vi "User Console View.vi"(8 "error in (no error)":errorcluster, 11 "View Model":T1) -> (0 "error out":errorcluster)   [LabVIEW 2017]
doc: "Provide processing user interaction with Elevator Controller by GUI controls."
uses:
  View Model/Controls/View Model.ctl
  Configuration/Controls/Config Model.ctl
  Configuration/Controls/Config Data.ctl
  Error Handler/Controls/Error Model.ctl
  Error Handler/Controls/Error Data.ctl
  Error Handler/Controls/Error Type.ctl
  View Model/Controls/Shared Model.ctl
  Elevator Controller/Controls/Elevator Model.ctl
  Elevator Controller/Controls/Elevator Location.ctl
  Elevator Controller/Controls/Elevator CMD Data.ctl
  Elevator Controller/Controls/Elevator Commands.ctl
  Elevator Controller/Controls/Elevator Overhead.ctl
  Elevator Controller/Controls/Elevator States.ctl
  Controls/User Console.ctl
panel:
  in  "Emergency":bool
  in  "1st Floor":bool
  in  "2nd Floor":bool
  in  "3rd Floor":bool
  in  "4th Floor":bool
  in  "Close Door":bool
  in  "Open Door":bool
  in  "Down 4":bool
  in  "Down 3":bool
  in  "Down 2":bool
  in  "Up 3":bool
  in  "Up 2":bool
  in  "Up 1":bool
  # "[Covers: UI1]"
  # "Floor Selection"
  # "Elevator Call"
  # "[Covers: UI2B]"
  # "[Covers: UI2A]"
  # "[Covers UI2A1]"
  # "[Covers UI2A2]"
  # "[Covers UI2B2]"
  # "by controls mechanical actions"
  # "[Covers: UI2C]"
  # "[Covers: UI2D]"
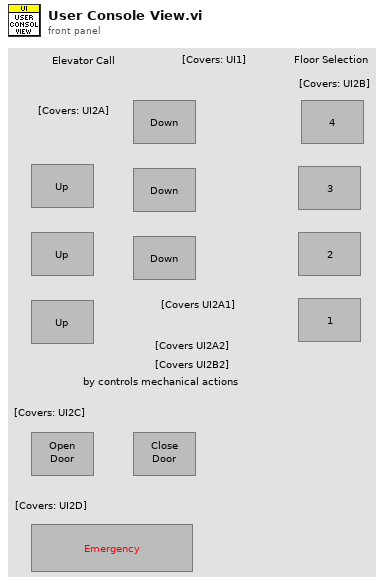
[diagram p1: front panel]
types:
  T1 = typedef "View Model.ctl" = cluster{"Config Model":T2, "Error Model":T3, "Shared Model":T4, "Elevator Model":T5}
  T2 = typedef "Config Model.ctl" = cluster{"Config Change":refnum<user-event>, "Config DVR":refnum<data-value>}
  T3 = typedef "Error Model.ctl" = cluster{"Error Event":refnum<user-event>}
  T4 = typedef "Shared Model.ctl" = cluster{"Stop Event":refnum<user-event>, "Stop DVR":refnum<data-value>}
  T5 = typedef "Elevator Model.ctl" = cluster{"Motion Change":refnum<user-event>, "Floor Change":refnum<user-event>, "Emergency Change":refnum<user-event>, "Direction Change":refnum<user-event>, "Door Position Change":refnum<user-event>, "Elevator CMD":refnum<user-event>, "Controller DVR":refnum<data-value>}
  T6 = typedef "User Console.ctl" = cluster{"Down 2":refnum<vi>, "Down 3":refnum<vi>, "Down 4":refnum<vi>, "Up 1":refnum<vi>, "Up 2":refnum<vi>, "Up 3":refnum<vi>, "1st Floor":refnum<vi>, "2nd Floor":refnum<vi>, "3rd Floor":refnum<vi>, "4th Floor":refnum<vi>, "Open Door":refnum<vi>, "Close Door":refnum<vi>, "Emergency":refnum<vi>}
  T7 = typedef "Elevator Commands.ctl" = enum16{"Go Up", "Go Down", "Go to Floor", "Open Doors", "Close Doors", "Emergency"}
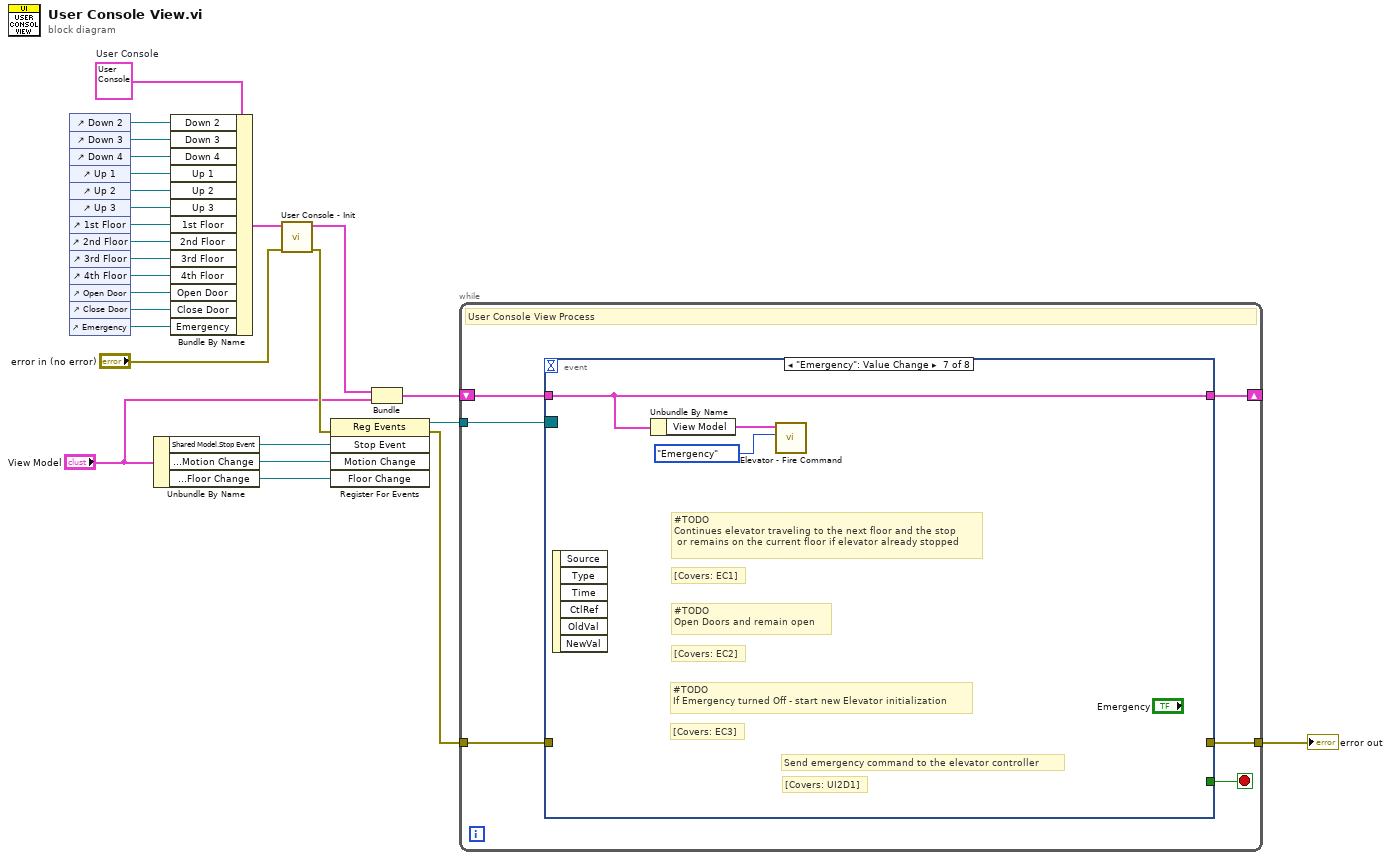
[diagram p0: block diagram]
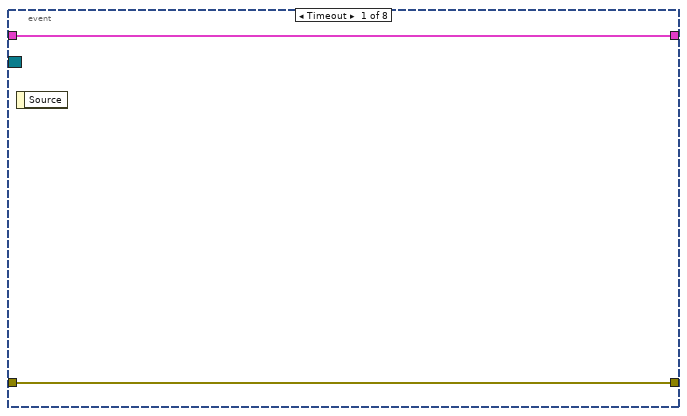
[diagram p2: hidden frame]
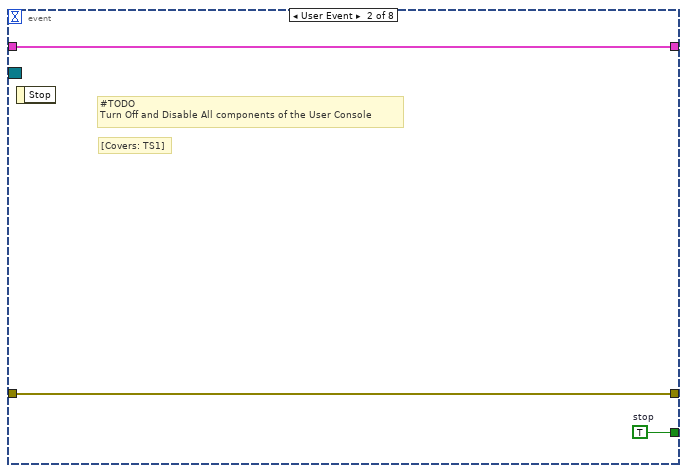
[diagram p3: hidden frame]
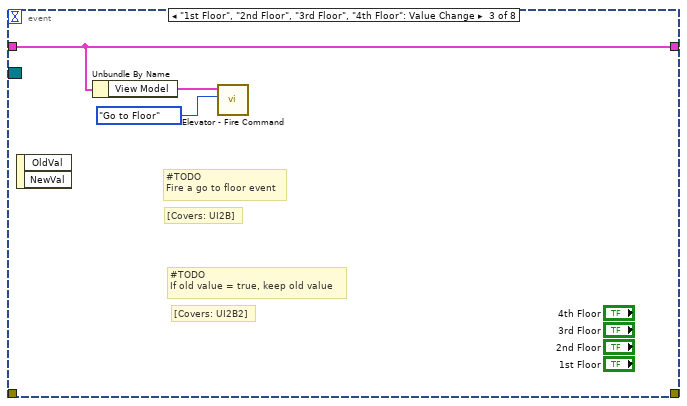
[diagram p4: hidden frame]
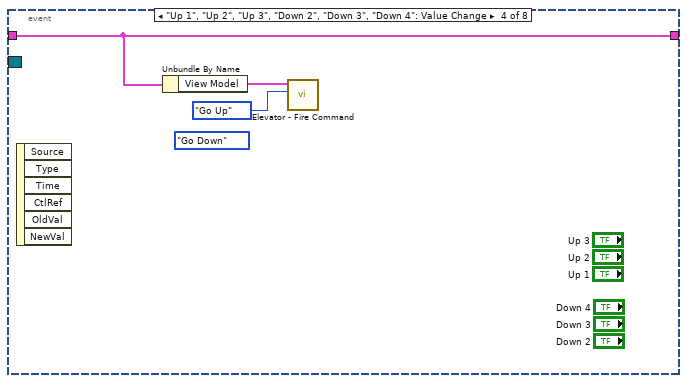
[diagram p5: hidden frame]
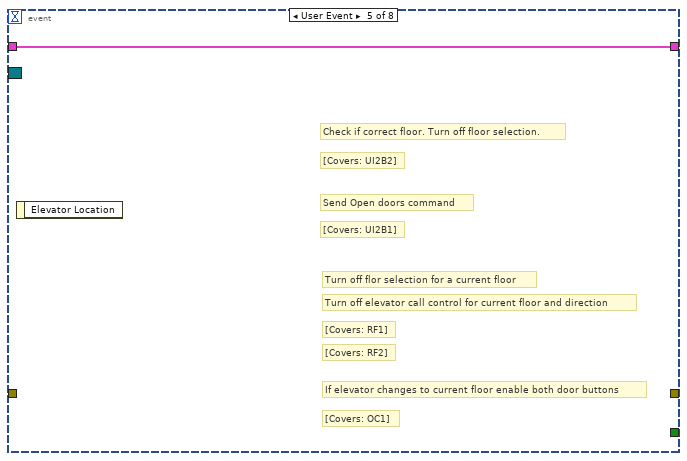
[diagram p6: hidden frame]
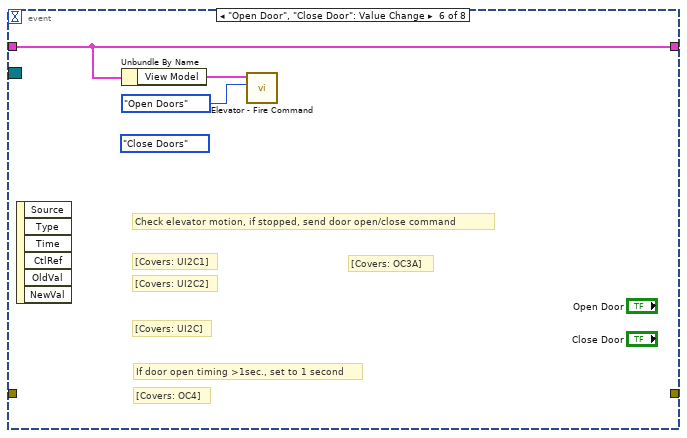
[diagram p7: hidden frame]
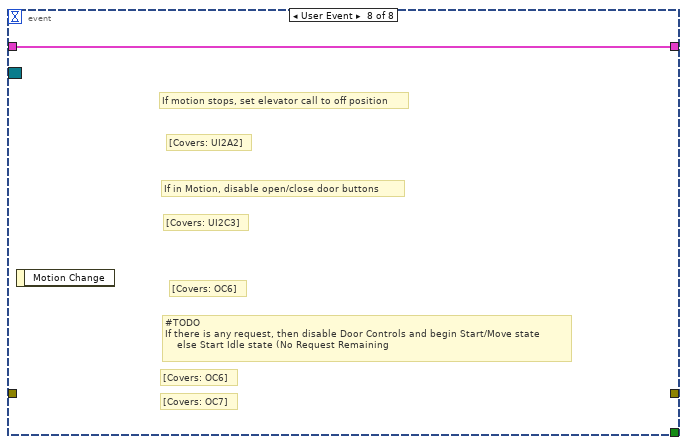
[diagram p8: hidden frame]
diagram:
  w21 = T6 {"Down 2"=refnum, "Down 3"=refnum, "Down 4"=refnum, "Up 1"=refnum, "Up 2"=refnum, "Up 3"=refnum, "1st Floor"=refnum, "2nd Floor"=refnum, "3rd Floor"=refnum, "4th Floor"=refnum, "Open Door"=refnum, "Close Door"=refnum, "Emergency"=refnum}  # User Console
  n1 = control-ref of="Down 2"() -> (w20:refnum<vi>)
  n2 = control-ref of="Down 3"() -> (w18:refnum<vi>)
  n3 = control-ref of="Down 4"() -> (w17:refnum<vi>)
  n4 = control-ref of="Up 1"() -> (w16:refnum<vi>)
  n5 = control-ref of="Up 2"() -> (w15:refnum<vi>)
  n6 = control-ref of="Up 3"() -> (w14:refnum<vi>)
  n7 = control-ref of="1st Floor"() -> (w13:refnum<vi>)
  n8 = control-ref of="2nd Floor"() -> (w12:refnum<vi>)
  n9 = control-ref of="3rd Floor"() -> (w11:refnum<vi>)
  n10 = control-ref of="4th Floor"() -> (w10:refnum<vi>)
  n11 = control-ref of="Open Door"() -> (w9:refnum<vi>)
  n12 = control-ref of="Close Door"() -> (w8:refnum<vi>)
  n13 = control-ref of="Emergency"() -> (w19:refnum<vi>)
  n14 = Unbundle By Name("View Model") -> ("Shared Model.Stop Event"=w26:refnum<user-event>, "Elevator Model.Motion Change"=w23:refnum<user-event>, "Elevator Model.Floor Change"=w22:refnum<user-event>)
  n15 = Bundle By Name(cluster=w21, "Down 2"=w20, "Down 3"=w18, "Down 4"=w17, "Up 1"=w16, "Up 2"=w15, "Up 3"=w14, "1st Floor"=w13, "2nd Floor"=w12, "3rd Floor"=w11, "4th Floor"=w10, "Open Door"=w9, "Close Door"=w8, "Emergency"=w19) -> (w7:T6)
  n16 = call "User Console - Init.vi"("error in (no error)"="error in (no error)", "User Console"=w7) -> ("error out"=w5:errorcluster, "User Console"=w2:T6)  [unwired: 8 in]
  n17 = register-events(error in=w5, w26, w23, w22) -> (reference out=w25:refnum<event-registration>, error out=w4:errorcluster)  [unwired: 1 in]
  n18 = Bundle("User Console"=w2, "View Model"="View Model") -> (w1:cluster{"User Console":T6, "View Model":T1})  [unwired: 1 in]
  n19 = while {
    tunnel: w25 -> [w32]
    tunnel: w4 -> [w30]
    tunnel: [w29] -> w24
    shift-right: [w27] -> _
    shift-left: w1 -> [w28]
    stop <- w31 stop-if-true
    # "User Console View Process"
    n20 = event shown="[6] \"Emergency\": Value Change" {
      selector: w32 -> [_ _ _ _ _ _ _ _]
      dyn-events: _ -> [_ _ _ _ _ _ _ _]
      timeout: _ -> [_ _ _ _ _ _ _ _]
      tunnel: [_ w37 _ _ _ _ _ _] -> w31
      tunnel: w30 -> [w34 w36 _ _ _ _ _ _]
      tunnel: [w34 w36 _ _ _ _ _ _] -> w29
      tunnel: w28 -> [w33 w35 w40 w41 w44 w45 w48 w51]
      tunnel: [w33 w35 w40 w41 w44 w45 w48 w51] -> w27
      event Timeout {
        n21 = event-data() -> ()  [unwired: 1 in, 1 out]
      }
      event User Event {
        w37 = TRUE  # stop
        # "[Covers: TS1]"
        # "#TODO\nTurn Off and Disable All components of the User Console"
        n22 = event-data() -> ()  [unwired: 1 in, 1 out]
      }
      event "1st Floor", "2nd Floor", "3rd Floor", "4th Floor": Value Change {
        # "[Covers: UI2B]"
        # "[Covers: UI2B2]"
        # "#TODO\nIf old value = true, keep old value"
        # "#TODO\nFire a go to floor event"
        n23 = event-data() -> ()  [unwired: 1 in, 2 out]
        n24 = Unbundle By Name(w40) -> ("View Model"=w39:T1)
        n25 = call "Elevator - Fire Command.vi"("Elevator Commands"=Elevator_Commands."Go to Floor", "View Model"=w39) -> ()  [unwired: 8 in, 2 out]
      }
      event "Up 1", "Up 2", "Up 3", "Down 2", "Down 3", "Down 4": Value Change {
        (unwired) Elevator_Commands."Go Down" ("Elevator Commands")
        n26 = event-data() -> ()  [unwired: 1 in, 6 out]
        n27 = Unbundle By Name(w41) -> ("View Model"=w43:T1)
        n28 = call "Elevator - Fire Command.vi"("Elevator Commands"=Elevator_Commands."Go Up", "View Model"=w43) -> ()  [unwired: 8 in, 2 out]
      }
      event User Event {
        # "[Covers: UI2B1]"
        # "Send Open doors command"
        # "Check if correct floor. Turn off floor selection."
        # "[Covers: UI2B2]"
        # "[Covers: OC1]"
        # "If elevator changes to current floor enable both door buttons"
        # "[Covers: RF2]"
        # "Turn off elevator call control for current floor and direction"
        # "[Covers: RF1]"
        # "Turn off flor selection for a current floor"
        n29 = event-data() -> ()  [unwired: 1 in, 1 out]
      }
      event "Open Door", "Close Door": Value Change {
        (unwired) Elevator_Commands."Close Doors" ("Elevator Commands")
        # "[Covers: OC3A]"
        # "[Covers: UI2C]"
        # "[Covers: UI2C2]"
        # "[Covers: UI2C1]"
        # "Check elevator motion, if stopped, send door open/close command"
        # "[Covers: OC4]"
        # "If door open timing >1sec., set to 1 second"
        n30 = event-data() -> ()  [unwired: 1 in, 6 out]
        n31 = Unbundle By Name(w45) -> ("View Model"=w47:T1)
        n32 = call "Elevator - Fire Command.vi"("Elevator Commands"=Elevator_Commands."Open Doors", "View Model"=w47) -> ()  [unwired: 8 in, 2 out]
      }
      event "Emergency": Value Change {
        # "[Covers: EC3]"
        # "#TODO\nIf Emergency turned Off - start new Elevator initialization"
        # "[Covers: EC2]"
        # "[Covers: EC1]"
        # "#TODO\nOpen Doors and remain open"
        # "#TODO\nContinues elevator traveling to the next floor and the stop\n or remains on the current floor if elevator already stopped"
        # "[Covers: UI2D1]"
        # "Send emergency command to the elevator controller"
        n33 = event-data() -> ()  [unwired: 1 in, 6 out]
        n34 = Unbundle By Name(w48) -> ("View Model"=w50:T1)
        n35 = call "Elevator - Fire Command.vi"("Elevator Commands"=Elevator_Commands."Emergency", "View Model"=w50) -> ()  [unwired: 8 in, 2 out]
      }
      event User Event {
        # "[Covers: OC7]"
        # "[Covers: OC6]"
        # "#TODO\nIf there is any request, then disable Door Controls and begin Start/Move state\n    else Start Idle state (No Request Remaining"
        # "[Covers: OC6]"
        # "[Covers: UI2C3]"
        # "If in Motion, disable open/close door buttons"
        # "[Covers: UI2A2]"
        # "If motion stops, set elevator call to off position"
        n36 = event-data() -> ()  [unwired: 1 in, 1 out]
      }
    }
  }
  "error out" <- w24
